vi "Offline_Analysis_FLDA_분석기_woF4.vi"(0 "LDA_matrix":path caption="LDA_matrix.txt", 1 "DIscard Channel Info":i32[](array[numeric]), 5 "Weight":path caption="weight.txt", 7 "Target_order.txt":path, 9 "mius_flash_order":path, 11 "Brain":path, 12 "피험자이름":string="홍길동", 13 "Save_path":string) -> ()   [LabVIEW 2014]
uses:
  <vilib>/Utility/file.llb/Read From Spreadsheet File (DBL).vi
  <vilib>/Analysis/Matrix/Numeric/Conversions/Array To Matrix - RA2.vi
  <vilib>/Analysis/Matrix/Numeric/Conversions/Array To Matrix - RA.vi
  <vilib>/Utility/file.llb/Read From Spreadsheet File (I64).vi
  <vilib>/Utility/file.llb/Write To Spreadsheet File (DBL).vi
  <vilib>/Utility/file.llb/Write To Spreadsheet File (I64).vi
  <vilib>/Utility/file.llb/Write To Spreadsheet File (string).vi
  <vilib>/Analysis/Matrix/NI_Matrix.lvlib
panel:
  out "ACC":i16
  in  "Channel selection":bool[](array[boolean])=[TRUE, TRUE, TRUE, TRUE, TRUE, TRUE, TRUE, TRUE, TRUE, TRUE, TRUE]
  out "Target_order":i64[](array[numeric])
  out "Selected_Target":i32[](array[numeric])
  out "Accuracy":i16[](array[numeric])
  in  "사용할 Parameter 갯수":i32=4
  out "error out":errorcluster
  in  "Random_num":i32=6
  in  "Flash_Repeat":i32=20
  in  "Frame_Length":i32=10
  in  "Sampling_Rate":dbl=250.0
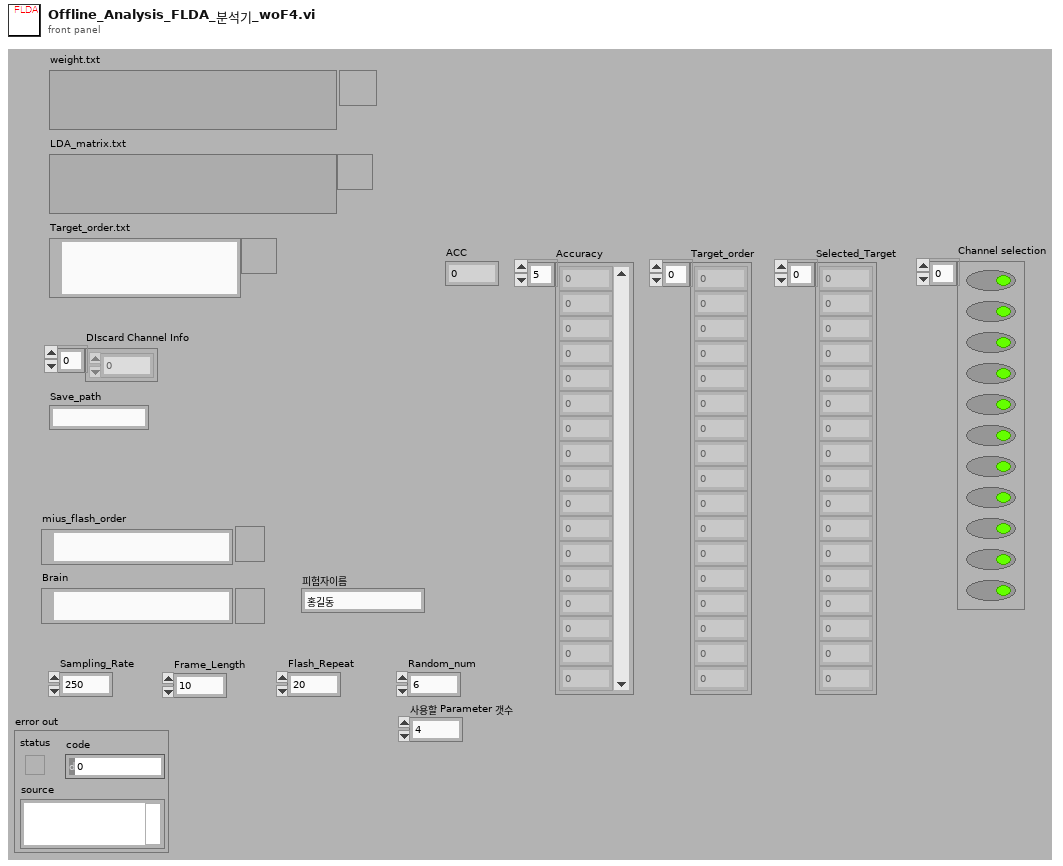
[diagram p1: front panel]
types:
  T1 = typedef "NI_Matrix.lvlib/RealMatrix.ctl" = dbl[][]
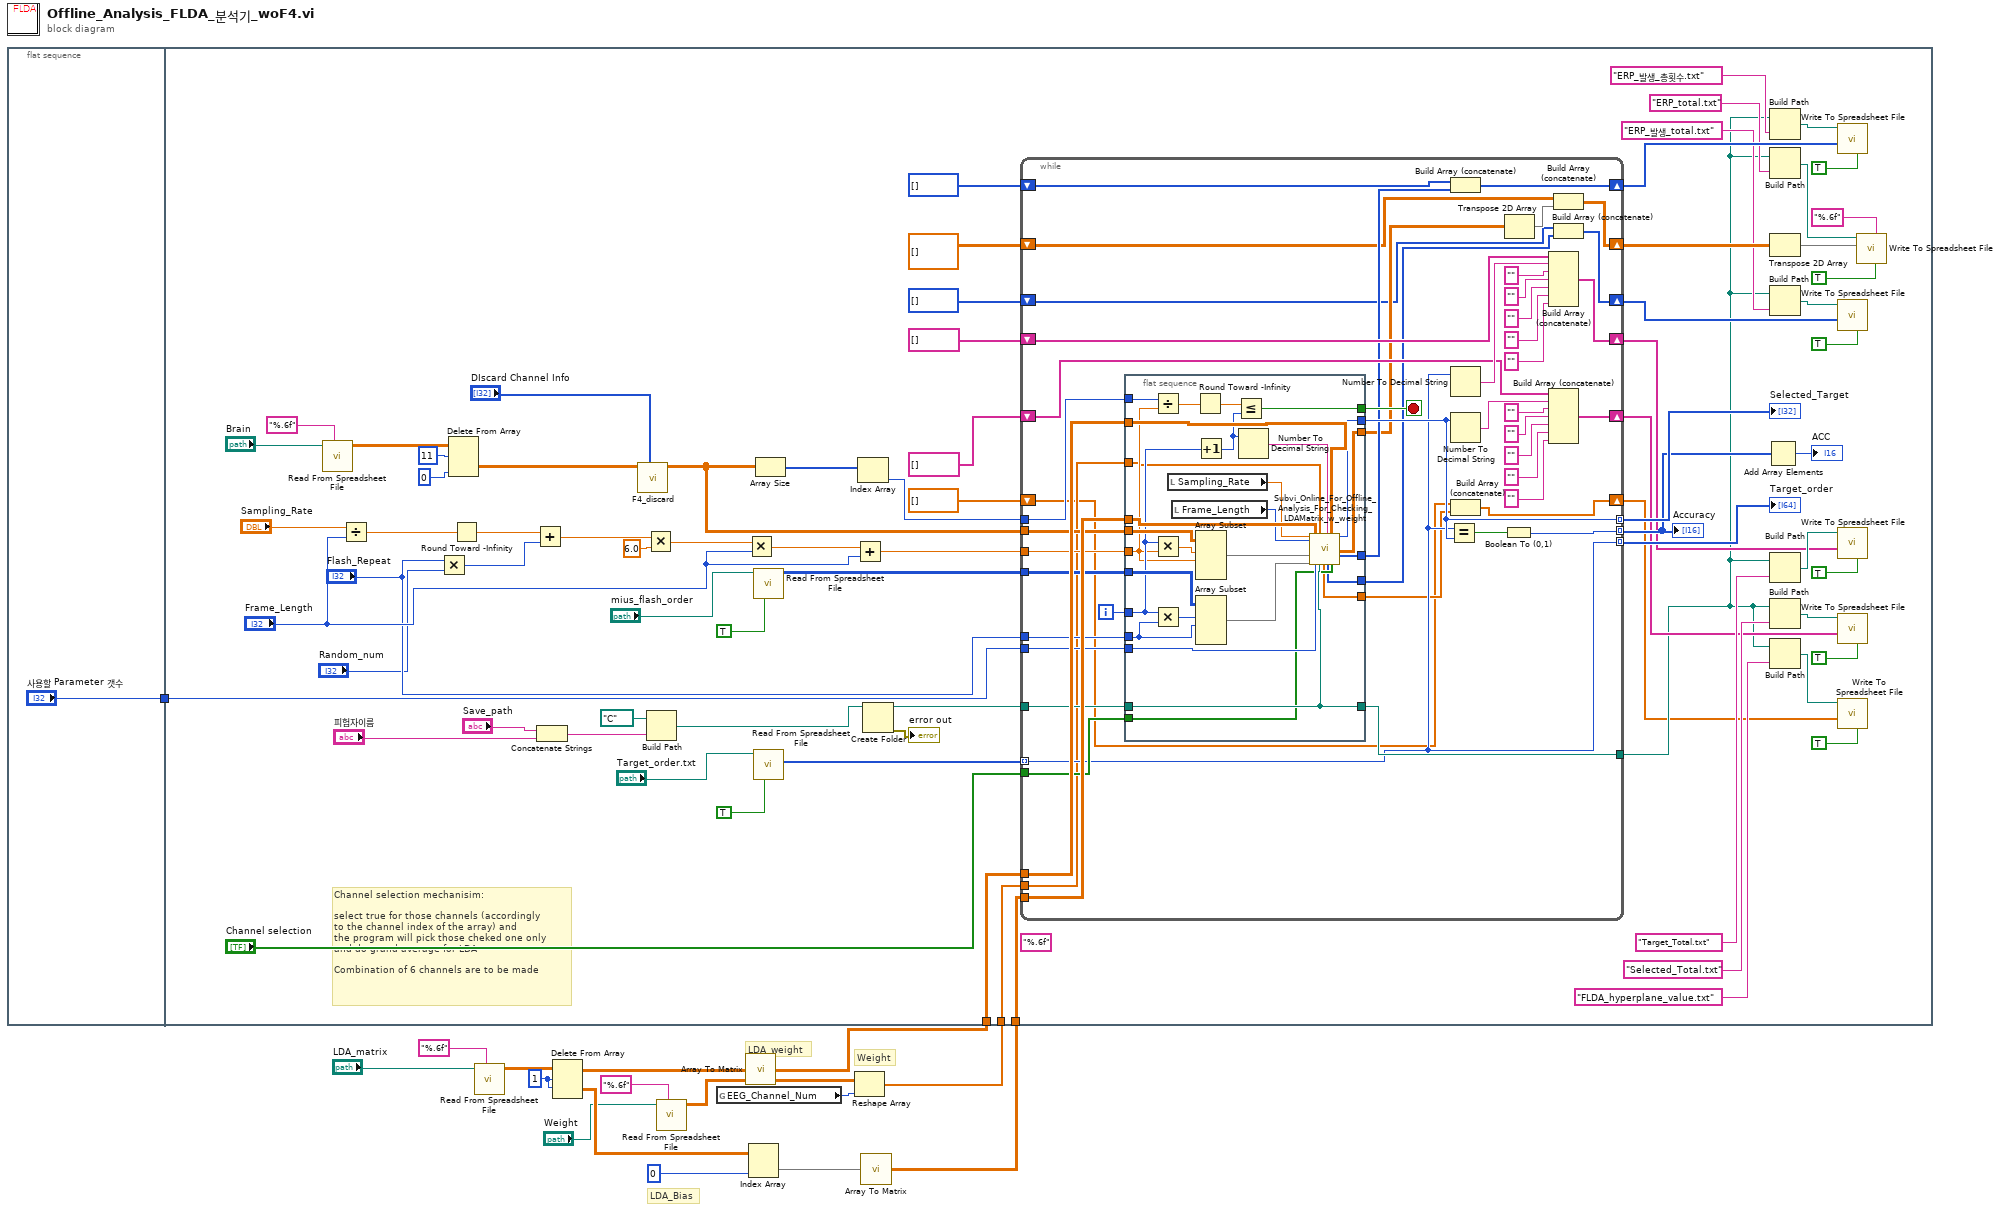
[diagram p0: block diagram]
diagram:
  w10 = 1 ("인덱스 (행)")
  # "LDA_Bias"
  # "LDA_weight"
  # "Weight"
  n1 = flat-sequence {
    tunnel: ["사용할 Parameter 갯수"] -> w16
    tunnel: w16 -> [w67]
    tunnel: w7 -> [w31]
    tunnel: w6 -> [w30]
    tunnel: w1 -> [w29]
    frame #0 {
    }
    frame #1 {
      (unwired) "%.6f" ("format (%.3f)")
      # "Channel selection mechanisim:\n\nselect true for those channels (accordingly\nto the channel index of the array) and \nthe program will pick those cheked one only\nand do grand average for LDA\n\nCombination of 6 channels are to be made"
      n2 = call-poly <vilib>:"Read From Spreadsheet File.vi"("format (%.3f)"="%.6f", "file path (dialog if empty)"="Brain") -> ("all rows"=w72:dbl[][])  [unwired: 5 in, 4 out]
      n3 = Divide(x="Sampling_Rate", y="Frame_Length") -> (x/y=w78:dbl)
      n4 = Multiply(x="Flash_Repeat", y="Random_num") -> (x*y=w81:i32)
      n5 = Delete From Array(array=w72, length=11 ("길이"), index (col)=0 ("비활성화된 인덱스 (열)")) -> (deleted portion=w28:dbl[][])  [unwired: 1 in, 1 out]
      n6 = Round Toward -Infinity(1:w78) -> (0:w80:dbl)
      n7 = Add(x=w80, y=w81) -> (x+y=w83:dbl)
      n8 = Concatenate Strings("Save_path", "피험자이름") -> (w21:string)
      n9 = call "F4_discard.vi"("DIscard Channel Info"="DIscard Channel Info", "Array"=w28) -> ("array w/ subset deleted"=w19:dbl[][])  [unwired: 9 in]
      n10 = Multiply(x=w83, y=6.0) -> (x*y=w85:dbl)
      n11 = Build Path(base path=path "C:/" ("path"), name or relative path=w21) -> (appended path=w90:path)
      n12 = Multiply(x=w85, y="Frame_Length") -> (x*y=w87:dbl)
      n13 = call-poly <vilib>:"Read From Spreadsheet File.vi"("transpose (no:F)"=TRUE, "file path (dialog if empty)"="mius_flash_order") -> ("all rows"=w74:i64[][])  [unwired: 5 in, 4 out]
      n14 = call-poly <vilib>:"Read From Spreadsheet File.vi"("transpose (no:F)"=TRUE, "file path (dialog if empty)"="Target_order.txt") -> ("first row"=w65:i64[])  [unwired: 5 in, 4 out]
      n15 = Array Size(array=w19) -> (size(s)=w75:i32[])
      n16 = Add(x=w87, y="Frame_Length") -> (x+y=w88:dbl)
      n17 = Index Array(array=w75) -> (element=w76:i32)  [unwired: 1 in]
      n18 = Create Folder(path (use dialog)=w90) -> (created path=w92:path, error out=→"error out":errorcluster)  [unwired: 2 in, 1 out]
      n19 = while {
        tunnel: w30 -> [w141]
        tunnel: w31 -> [w140]
        tunnel: w19 -> [w138]
        tunnel: w74 -> [w137]
        tunnel: w76 -> [w139]
        tunnel: w88 -> [w135]
        tunnel: "Flash_Repeat" -> [w136]
        tunnel: w92 -> [w134]
        tunnel: w67 -> [w133]
        tunnel: w65 -> [w111] mode=indexing
        tunnel: [w131] -> w53 mode=indexing
        tunnel: [w111] -> w62 mode=indexing
        tunnel: [w112] -> w63 mode=indexing
        tunnel: "Channel selection" -> [w128]
        tunnel: [w127] -> w23
        shift-right: [w114] -> w47
        shift-left: string[] [] -> [w113]
        shift-right: [w110] -> w46
        shift-left: string[] [] -> [w109]
        shift-right: [w107] -> w44
        shift-left: i16[] [] -> [w106]
        shift-right: [w103] -> w39
        shift-left: dbl[][] [] -> [w102]
        shift-right: [w100] -> w32
        shift-left: i16[] [] -> [w99]
        tunnel: w29 -> [w98]
        shift-right: [w95] -> w22
        shift-left: dbl[] [] -> [w96]
        i -> [w130]
        stop <- w129 stop-if-true
        n20 = flat-sequence {
          tunnel: [w169] -> w108
          tunnel: [w168] -> w127
          tunnel: w98 -> [w144]
          tunnel: [w145] -> w101
          tunnel: [w147] -> w105
          tunnel: w128 -> [w148]
          tunnel: [w149] -> w112
          tunnel: w133 -> [w150]
          tunnel: w134 -> [w168]
          tunnel: w135 -> [w156]
          tunnel: w130 -> [w157]
          tunnel: w136 -> [w158]
          tunnel: w137 -> [w160]
          tunnel: w138 -> [w163]
          tunnel: [w164] -> w129
          tunnel: w139 -> [w165]
          tunnel: w140 -> [w166]
          tunnel: w141 -> [w167]
          tunnel: [w142] -> w97
          frame #0 {
            n21 = Divide(x=w165, y=w156) -> (x/y=w155:dbl)
            n22 = Multiply(x=w157, y=w156) -> (x*y=w162:dbl)
            n23 = Multiply(x=w157, y=w158) -> (x*y=w159:i32)
            n24 = local read "Sampling_Rate"() -> (w153:dbl)
            n25 = local read "Frame_Length"() -> (w152:i32)
            n26 = Round Toward -Infinity(1:w155) -> (0:w154:dbl)
            n27 = Increment(x=w157) -> (x+1=w151:i32)
            n28 = Array Subset(array=w163, index (row)=w162, length (row)=w156) -> (w161:dbl[][])  [unwired: 2 in]
            n29 = Array Subset(array=w160, index (row)=w159, length (row)=w158) -> (w143:i64[][])  [unwired: 2 in]
            n30 = Less Or Equal?(x=w154, y=w151) -> (x <= y?=w164:bool)
            n31 = Number To Decimal String(number=w151) -> (decimal integer string=w146:string)  [unwired: 1 in]
            n32 = call "Subvi_Online_For_Offline_Analysis_For_Checking_LDAMatrix_w_weight.vi"("rate"=w153, "samples per channel"=w152, "Brain_data_source"=w161, "Target_Flash_Order"=w143, "Value"=w167, "사용할 Parameter 갯수"=w150, "Weight"=w144, "Path"=w168, "Number"=w146, "Matrix"=w166, "Channel selection"=w148) -> ("Array"=w142:dbl[], "자극별 ERP 발생여부"=w145:i16[], "output-0~8"=w149:i32, "ERP_all"=w147:dbl[][], "자극별 ERP 발생 총 횟수"=w169:i16[])  [unwired: 12 in]
          }
        }
        n33 = Equal?(x=w111, y=w112) -> (x = y?=w132:bool)
        n34 = Build Array (concatenate)(w106, w108) -> (w107:i16[])
        n35 = Number To Decimal String(number=w111) -> (decimal integer string=w126:string)  [unwired: 1 in]
        n36 = Number To Decimal String(number=w112) -> (decimal integer string=w120:string)  [unwired: 1 in]
        n37 = Build Array (concatenate)(w96, w97) -> (w95:dbl[])
        n38 = Boolean To (0,1)(Boolean=w132) -> (0, 1=w131:i16)
        n39 = Transpose 2D Array(2D array=w105) -> (transposed array=w104:dbl[][])
        n40 = Build Array (concatenate)(w109, w126, "" ("element"), "" ("element"), "" ("element"), "" ("element"), "" ("element")) -> (w110:string[])
        n41 = Build Array (concatenate)(w113, w120, "" ("element"), "" ("element"), "" ("element"), "" ("element"), "" ("element")) -> (w114:string[])
        n42 = Build Array (concatenate)(w102, w104) -> (w103:dbl[][])
        n43 = Build Array (concatenate)(w99, w101) -> (w100:i16[])
      }
      "Accuracy" <- w53
      "Selected_Target" <- w63
      "Target_order" <- w62
      n44 = Add Array Elements(numeric array=w53) -> (sum=→"ACC":i16)
      n45 = Build Path(base path=w23, name or relative path="ERP_발생_총횟수.txt") -> (appended path=w57:path)
      n46 = Build Path(base path=w23, name or relative path="ERP_total.txt") -> (appended path=w40:path)
      n47 = Transpose 2D Array(2D array=w39) -> (transposed array=w37:dbl[][])
      n48 = Build Path(base path=w23, name or relative path="ERP_발생_total.txt") -> (appended path=w34:path)
      n49 = Build Path(base path=w23, name or relative path="Target_Total.txt") -> (appended path=w55:path)
      n50 = Build Path(base path=w23, name or relative path="Selected_Total.txt") -> (appended path=w49:path)
      n51 = Build Path(base path=w23, name or relative path="FLDA_hyperplane_value.txt") -> (appended path=w25:path)
      n52 = call-poly <vilib>:"Write To Spreadsheet File.vi"("transpose? (no:F)"=TRUE, "1D data"=w44, "file path (dialog if empty)"=w57) -> ()  [unwired: 5 in, 1 out]
      n53 = call-poly <vilib>:"Write To Spreadsheet File.vi"("transpose? (no:F)"=TRUE, "1D data"=w32, "file path (dialog if empty)"=w34) -> ()  [unwired: 5 in, 1 out]
      n54 = call-poly <vilib>:"Write To Spreadsheet File.vi"("transpose? (no:F)"=TRUE, "1D data"=w46, "file path (dialog if empty)"=w55) -> ()  [unwired: 5 in, 1 out]
      n55 = call-poly <vilib>:"Write To Spreadsheet File.vi"("transpose? (no:F)"=TRUE, "1D data"=w47, "file path (dialog if empty)"=w49) -> ()  [unwired: 5 in, 1 out]
      n56 = call-poly <vilib>:"Write To Spreadsheet File.vi"("transpose? (no:F)"=TRUE, "1D data"=w22, "file path (dialog if empty)"=w25) -> ()  [unwired: 5 in, 1 out]
      n57 = call-poly <vilib>:"Write To Spreadsheet File.vi"("transpose? (no:F)"=TRUE, "format (%.3f)"="%.6f", "2D data"=w37, "file path (dialog if empty)"=w40) -> ()  [unwired: 4 in, 1 out]
    }
  }
  n58 = call-poly <vilib>:"Read From Spreadsheet File.vi"("format (%.3f)"="%.6f", "file path (dialog if empty)"="LDA_matrix") -> ("all rows"=w8:dbl[][])  [unwired: 5 in, 4 out]
  n59 = Delete From Array(array=w8, length=w10, index (row)=w10) -> (deleted portion=w13:dbl[][], array with subset deleted=w12:dbl[][])  [unwired: 1 in]
  n60 = call-poly <vilib>:"Read From Spreadsheet File.vi"("format (%.3f)"="%.6f", "file path (dialog if empty)"="Weight") -> ("all rows"=w3:dbl[][])  [unwired: 5 in, 4 out]
  n61 = global read "Control_Panel_정리.vi" "EEG_Channel_Num"() -> (w2:i32)
  n62 = call-poly <vilib>:"Array To Matrix.vi"("Real 2D Array"=w12) -> ("Real Matrix"=w7:T1)
  n63 = Index Array(array=w13, index (col)=0 ("인덱스")) -> (element=w11:dbl[])  [unwired: 1 in]
  n64 = Reshape Array(w3, w2) -> (w1:dbl[])
  n65 = call-poly <vilib>:"Array To Matrix.vi"("Real 1D Array"=w11) -> ("Real Matrix (Column Vector)"=w6:T1)
